vi "Get Settings Name.vi"(8 "error in (no error)":errorcluster {"code" format="Error %.0f"}, 11 "VIDoc Settings - Confluence In":refnum<class "VIDoc Settings - Confluence.lvclass">) -> (0 "error out":errorcluster {"code" format="Error %.0f"}, 2 "Name":string, 3 "VIDoc Settings - Confluence Out":refnum<class "VIDoc Settings - Confluence.lvclass">)   [LabVIEW 2023, in "VIDoc Printer - Confluence.lvlib" / "VIDoc Settings - Confluence.lvclass"]
uses:
  VIDoc Settings - Confluence.lvclass
  VIDoc Settings - Confluence.lvclass/VIDoc Settings - Confluence.ctl
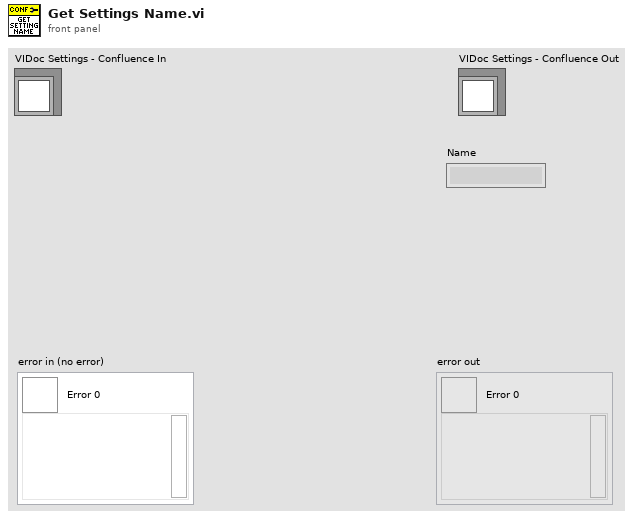
[diagram p1: front panel]
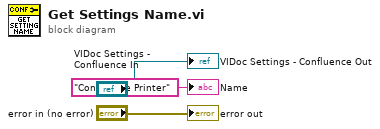
[diagram p0: block diagram]
diagram:
  "error out" <- "error in (no error)"
  "VIDoc Settings - Confluence Out" <- "VIDoc Settings - Confluence In"
  "Name" <- "Confluence Printer" ("Name")
